vi "Command_Joint_Angles_array.vi"(4 "Mode":T2(ring), 5 "node":string, 6 "error in":errorcluster, 7 "Arm Angles (degrees)":dbl[](array[numeric]), 9 "Side":T3) -> (0 "error out":errorcluster, 3 "JointCommand":T1={"Mode"=enum."Position", "Arm Angles"=[], "Angle Names"=["_s0", "_s1", "_e0", "_e1", "_w0", "_w1", "_w2"]})   [LabVIEW 2013]
uses:
  ROS/Code/SubVIs/BaxterSide.ctl
  ROS/RosMessages/Clusters/JointCommand.ctl
  Read_Joint_States_A.vi
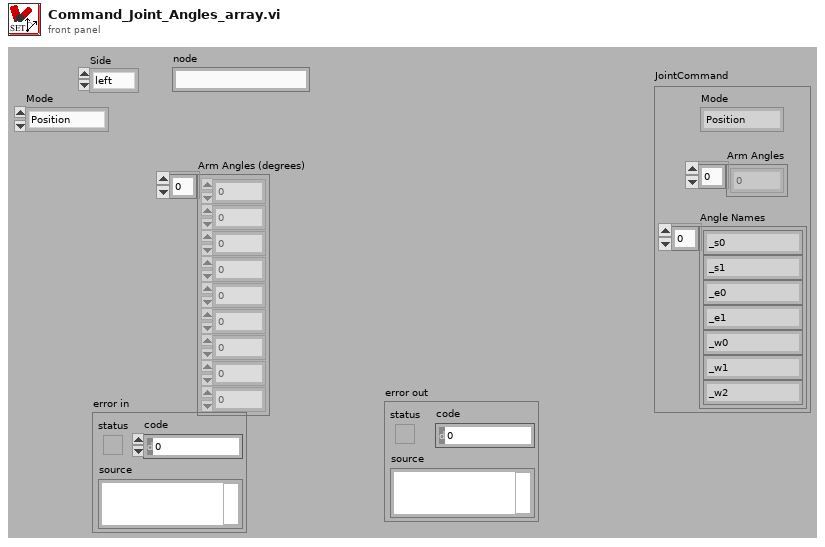
[diagram p1: front panel]
types:
  T1 = typedef "JointCommand.ctl" = cluster{"Mode":enum32{"", "Position", "Velocity", "Effort"}, "Arm Angles":dbl[], "Angle Names":string[]}
  T2 = enum32{"Position", "Velocity", "Effort", "Pause", "Repeat"}
  T3 = typedef "BaxterSide.ctl" = enum16{"left", "right"}
  T4 = enum16{"big-endian, network order", "native, host order", "little-endian"}
  T5 = typedef "_ROSControl.ctl" = cluster{"topic port":u16, "Node":string, "topic":string, "type":string, "node port":u32, "error ":errorcluster, "Direction":T6, "APIs":string[]}
  T6 = typedef "_ROSDirection.ctl" = enum16{"Node", "Publisher", "Subscriber", "Service Client"}
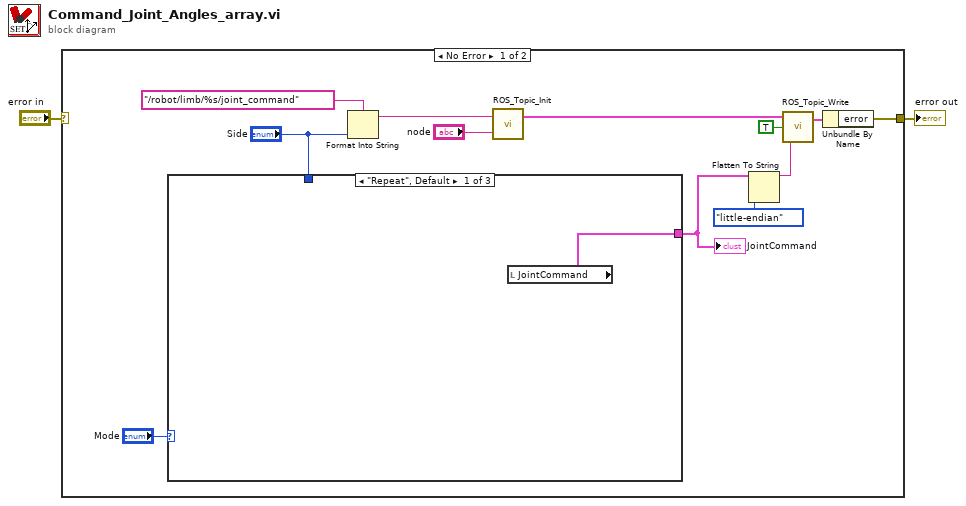
[diagram p0: block diagram]
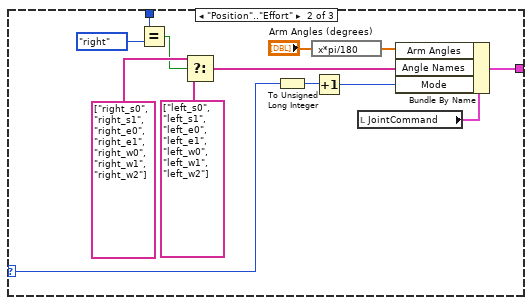
[diagram p2: hidden frame]
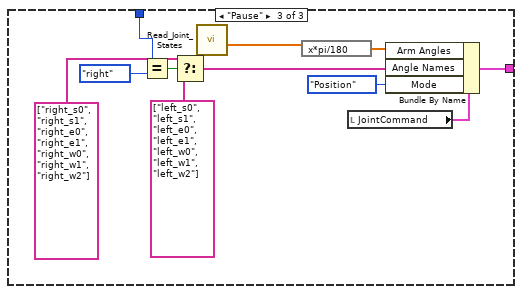
[diagram p3: hidden frame]
diagram:
  n1 = case shown="No Error" "error in" {
    selector: "error in" -> [_ w40]
    tunnel: [w14 w40] -> w2
    frame No Error {
      n2 = case shown="\"Repeat\", Default" "Mode" {
        selector: "Mode" -> [_ w17 _]
        tunnel: "Side" -> [_ w26 w39]
        tunnel: [w15 w16 w32] -> w4
        frame "Repeat", Default {
          n3 = local read "JointCommand"() -> (w15:T1)
        }
        frame "Position".."Effort" {
          n4 = Equal?(x=w26, y=BaxterSide."right") -> (x = y?=w23:bool)
          n5 = Select(t=string[] ["right_s0", "right_s1", "right_e0", "right_e1", "right_w0", "right_w1", "right_w2"] ("Angle Names"), s=w23, f=string[] ["left_s0", "left_s1", "left_e0", "left_e1", "left_w0", "left_w1", "left_w2"] ("Angle Names")) -> (s? t:f=w21:string[])
          n6 = To Unsigned Long Integer(number=w17) -> (unsigned 32bit integer=w19:u32)
          n7 = expression code="x*pi/180"("Arm Angles (degrees)") -> (w20:dbl[])
          n8 = Increment(x=w19) -> (x+1=w27:u32)
          n9 = local read "JointCommand"() -> (w18:T1)
          n10 = Bundle By Name(cluster=w18, "Arm Angles"=w20, "Angle Names"=w21, "Mode"=w27) -> (w16:T1)
        }
        frame "Pause" {
          n11 = Equal?(x=w39, y=BaxterSide."right") -> (x = y?=w36:bool)
          n12 = Select(t=string[] ["right_s0", "right_s1", "right_e0", "right_e1", "right_w0", "right_w1", "right_w2"] ("Angle Names"), s=w36, f=string[] ["left_s0", "left_s1", "left_e0", "left_e1", "left_w0", "left_w1", "left_w2"] ("Angle Names")) -> (s? t:f=w34:string[])
          n13 = call-poly "Read_Joint_States.vi"() -> ("right Positions"=w30:dbl[])  [unwired: 5 in, 3 out]
          n14 = expression code="x*pi/180"(w30) -> (w33:dbl[])
          n15 = local read "JointCommand"() -> (w31:T1)
          n16 = Bundle By Name(cluster=w31, "Arm Angles"=w33, "Angle Names"=w34, "Mode"=enum32{"", "Position", "Velocity", "Effort"}."Position") -> (w32:T1)
        }
      }
      "JointCommand" <- w4
      n17 = Format Into String(format string="/robot/limb/%s/joint_command" ("topic"), "Side") -> (resulting string=w12:string)  [unwired: 2 in, 1 out]
      n18 = call "ROS_Topic_Init.vi"("node"="node", "topic"=w12) -> ("ROS out"=w11:T5)  [unwired: 1 in]
      n19 = Flatten To String(anything=w4, byte order (0:big-endian, network order)=T4."little-endian") -> (data string=w5:string)  [unwired: 2 in, 2 out]
      n20 = call "ROS_Topic_Write.vi"("Msg in"=w5, "Continuous?"=TRUE, "ROS in"=w11) -> ("ROS out"=w10:T5)  [unwired: 1 in]
      n21 = Unbundle By Name(w10) -> ("error"=w14:errorcluster)
    }
    frame Error {
    }
  }
  "error out" <- w2
